vi "ParseSysexCapabilityQuery.vi"(8 "error in":errorcluster, 11 "Sysex Message":u8[](array[numeric]) format="%x") -> (0 "error out":errorcluster, 1 "IsValidSysex":bool, 3 "Board Pins":T1[](array[typedef]) {"Index"."DigitalIndex" step=1 format="D%d"; "Index"."AnalogIndex" min=0.0 step=1.0 format="A%#.0g"})   [LabVIEW 2020, in "FirmataClient.lvlib"]
doc: "Parse a message according to the Firmata Protocol Requirements. \n- https://github.com/firmata/protocol\n- https://github.com/firmata/protocol/blob/master/protocol.md"
uses:
  FirmataClient.lvlib
  controls/PinModesListData.ctl
  controls/PinModeData.ctl
  controls/FirmataPinModes.ctl
  controls/FGV-Mode.ctl
  controls/FirmataProtocolConstants.ctl
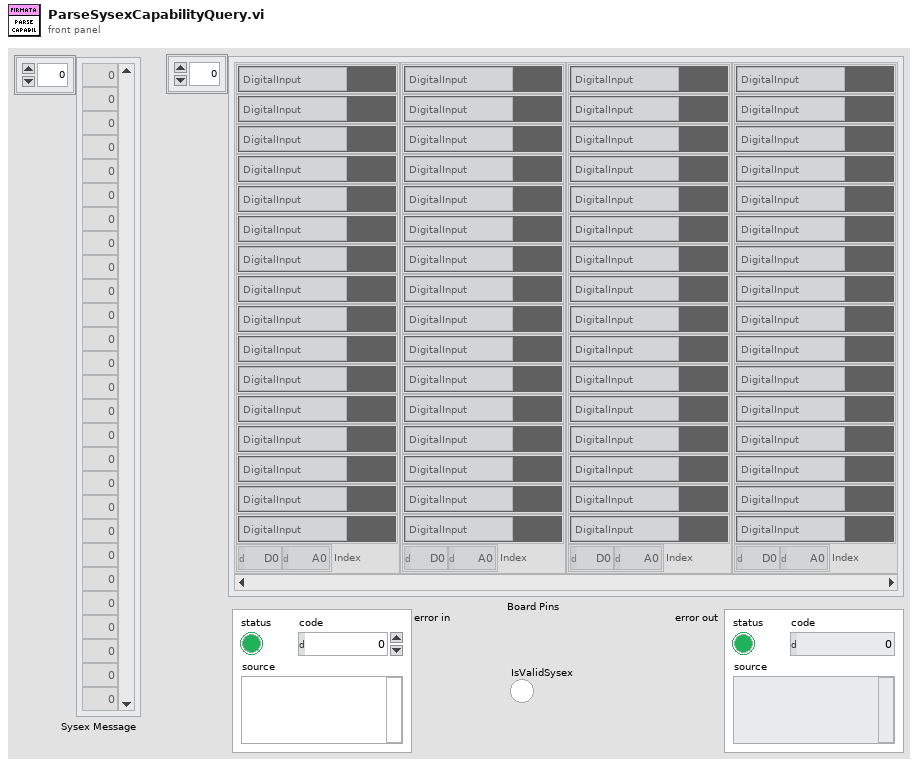
[diagram p1: front panel]
types:
  T1 = typedef "FirmataClient.lvlib/PinModesListData.ctl" = cluster{"DigitalInputMode":T2, "DigitalOutputMode":T2, "AnalogInputMode":T2, "PWMMode":T2, "ServoMode":T2, "ShiftMode":T2, "I2CMode":T2, "OneWireMode":T2, "StepperMode":T2, "EncoderMode":T2, "SerialMode":T2, "InputPullupMode":T2, "Ext.SPIMode":T2, "Ext.SonarMode":T2, "Ext.ToneMode":T2, "Ext.DHTMode":T2, "Index":cluster{"DigitalIndex":u16, "AnalogIndex":dbl}}
  T2 = typedef "FirmataClient.lvlib/PinModeData.ctl" = cluster{"Resolution":u8, "btn":bool, "PinMode":T3}
  T3 = typedef "FirmataClient.lvlib/FirmataPinModes.ctl" = enum16{"DigitalInput", "DigitalOutput", "AnalogInput", "PWM", "Servo", "Shift", "I2C", "OneWire", "Stepper", "Encoder", "Serial", "InputPullup", "Extended.SPI", "Extended.Sonar", "Extended.Tone", "Extended.DHT"}
  T4 = typedef "FirmataClient.lvlib/FirmataProtocolConstants.ctl" = u16
  T5 = typedef "FirmataClient.lvlib/FGV-Mode.ctl" = enum16{"Load Comport", "Load Board Capabilities", "Read"}
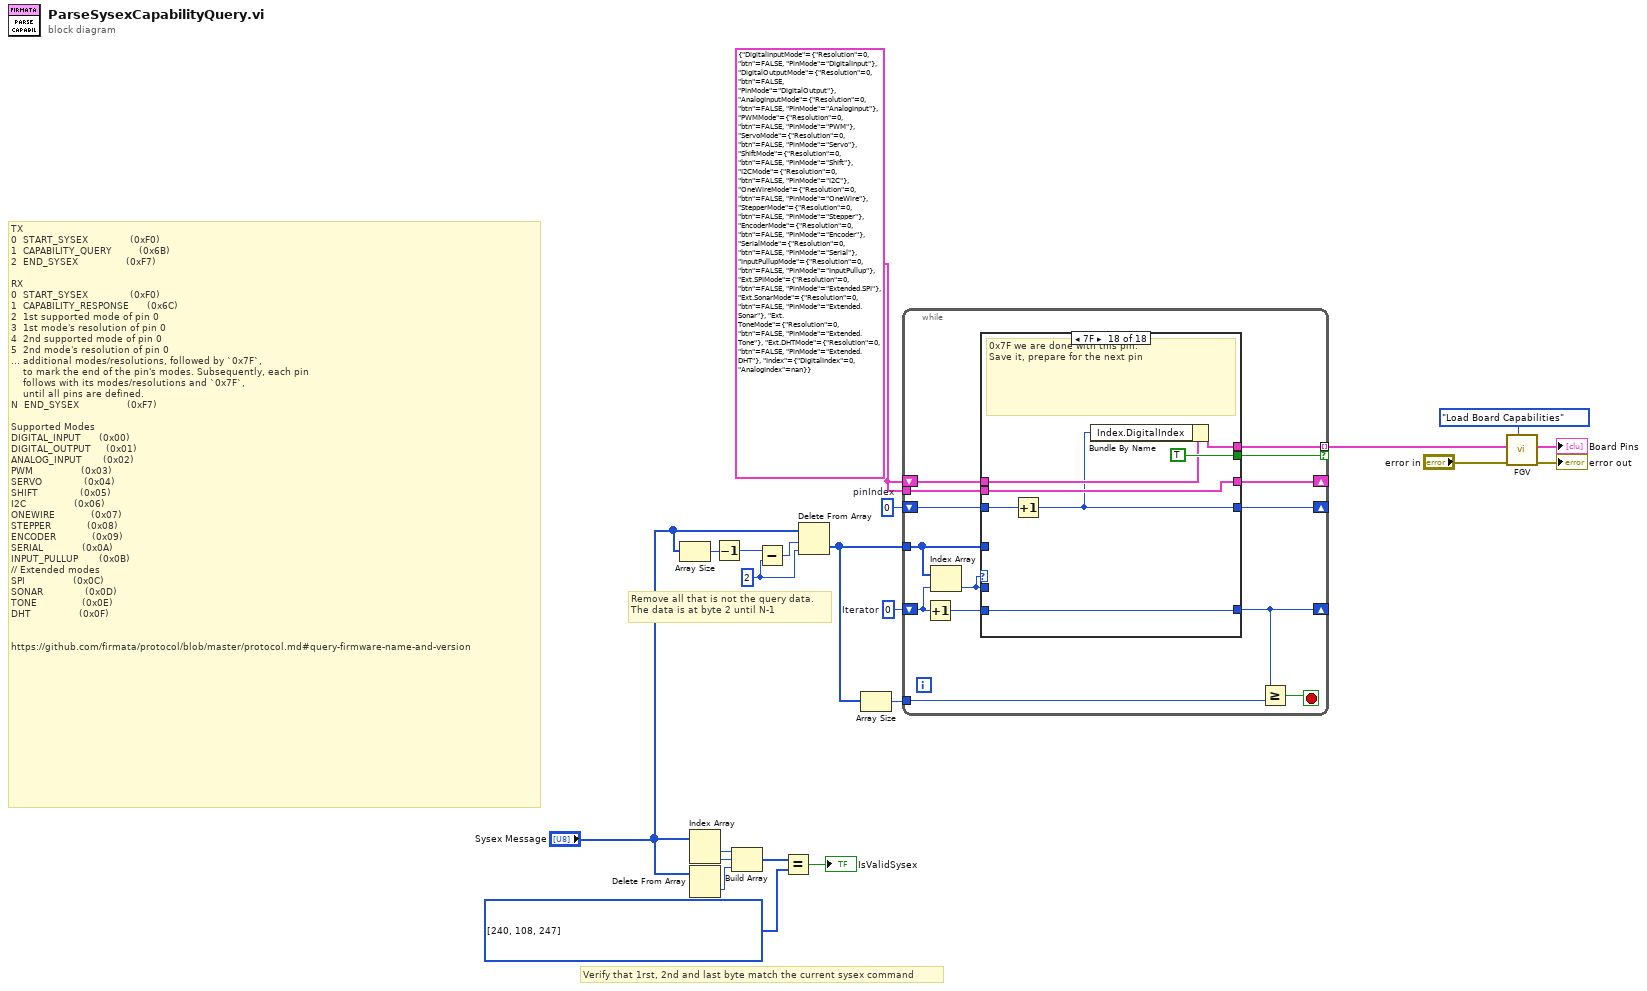
[diagram p0: block diagram]
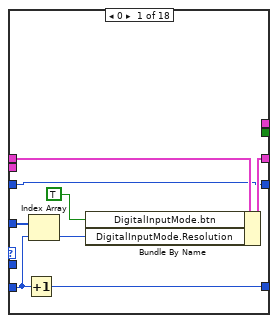
[diagram p2: hidden frame]
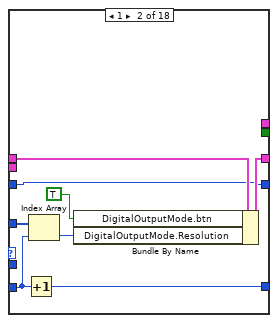
[diagram p3: hidden frame]
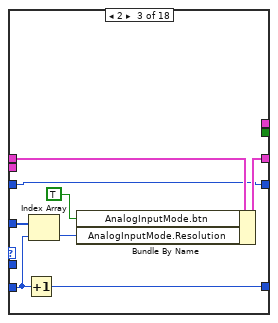
[diagram p4: hidden frame]
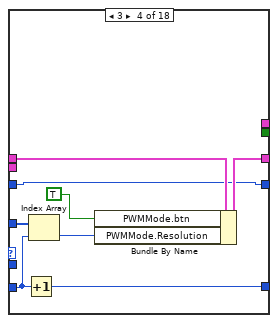
[diagram p5: hidden frame]
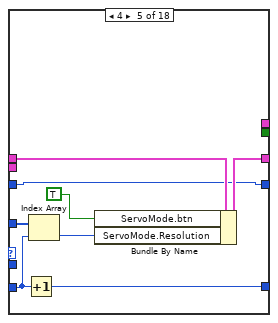
[diagram p6: hidden frame]
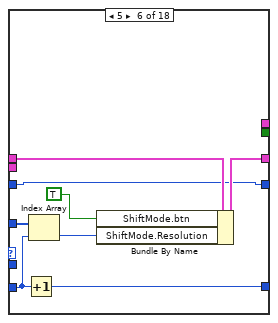
[diagram p7: hidden frame]
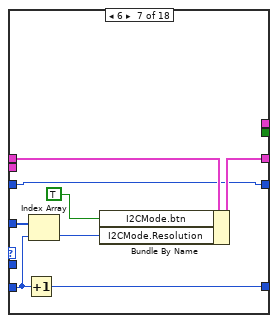
[diagram p8: hidden frame]
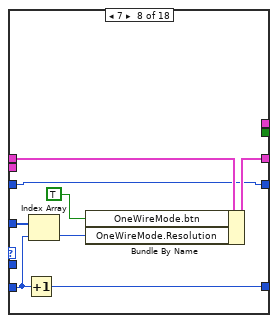
[diagram p9: hidden frame]
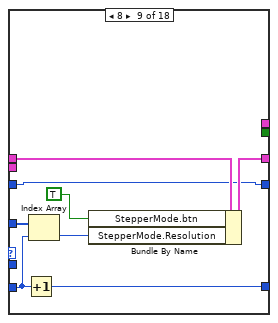
[diagram p10: hidden frame]
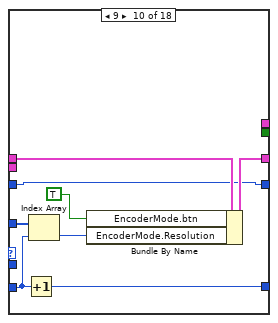
[diagram p11: hidden frame]
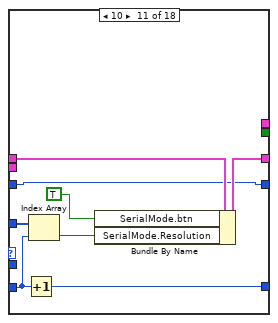
[diagram p12: hidden frame]
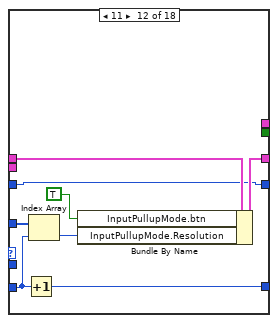
[diagram p13: hidden frame]
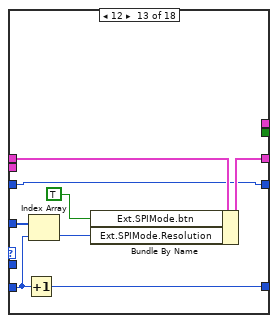
[diagram p14: hidden frame]
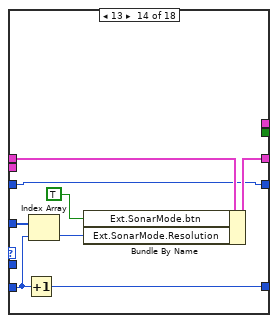
[diagram p15: hidden frame]
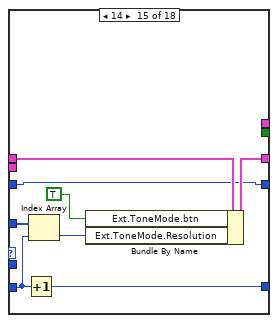
[diagram p16: hidden frame]
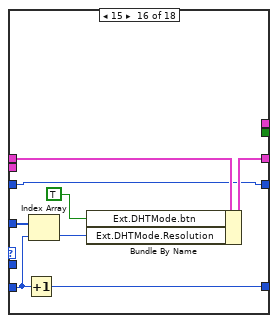
[diagram p17: hidden frame]
diagram:
  w3 = 0  # pinIndex
  w4 = T4[] [240, 108, 247] items=["ANALOG_IO_MESSAGE"=224, "DIGITAL_IO_MESSAGE"=144, "REPORT_ANALOG_PIN"=192, "REPORT_DIGITAL_PORT"=208, "START_SYSEX"=240, "END_SYSEX"=247, "SET_PIN_MODE"=244, "SET_DIGITAL_PIN_VALUE"=245, "PROTOCOL_VERSION"=249, "SYSTEM_RESET"=255, "SYSEX.EXTENDED_ID"=0, "SYSEX.RESERVED_USER_COMMANDs"=1, "SYSEX.ANALOG_MAPPING_QUERY"=105, "SYSEX.ANALOG_MAPPING_RESPONSE"=106, "SYSEX.CAPABILITY_QUERY"=107, "SYSEX.CAPABILITY_RESPONSE"=108, "SYSEX.PIN_STATE_QUERY"=109, "SYSEX.PIN_STATE_RESPONSE"=110, "SYSEX.REPORT_FIRMWARE"=121, "SYSEX.EXTENDED_ANALOG"=111, "SYSEX.STRING_DATA"=113, "SYSEX.REALTIME"=127, "SYSEX.NON_REALTIME"=126, "SYSEX.SAMPLING_INTERVAL"=122]
  w10 = 0  # Iterator
  w11 = T1 {"DigitalInputMode"={"Resolution"=0, "btn"=FALSE, "PinMode"=enum."DigitalInput"}, "DigitalOutputMode"={"Resolution"=0, "btn"=FALSE, "PinMode"=enum."DigitalOutput"}, "AnalogInputMode"={"Resolution"=0, "btn"=FALSE, "PinMode"=enum."AnalogInput"}, "PWMMode"={"Resolution"=0, "btn"=FALSE, "PinMode"=enum."PWM"}, "ServoMode"={"Resolution"=0, "btn"=FALSE, "PinMode"=enum."Servo"}, "ShiftMode"={"Resolution"=0, "btn"=FALSE, "PinMode"=enum."Shift"}, "I2CMode"={"Resolution"=0, "btn"=FALSE, "PinMode"=enum."I2C"}, "OneWireMode"={"Resolution"=0, "btn"=FALSE, "PinMode"=enum."OneWire"}, "StepperMode"={"Resolution"=0, "btn"=FALSE, "PinMode"=enum."Stepper"}, "EncoderMode"={"Resolution"=0, "btn"=FALSE, "PinMode"=enum."Encoder"}, "SerialMode"={"Resolution"=0, "btn"=FALSE, "PinMode"=enum."Serial"}, "InputPullupMode"={"Resolution"=0, "btn"=FALSE, "PinMode"=enum."InputPullup"}, "Ext.SPIMode"={"Resolution"=0, "btn"=FALSE, "PinMode"=enum."Extended.SPI"}, "Ext.SonarMode"={"Resolution"=0, "btn"=FALSE, "PinMode"=enum."Extended.Sonar"}, "Ext.ToneMode"={"Resolution"=0, "btn"=FALSE, "PinMode"=enum."Extended.Tone"}, "Ext.DHTMode"={"Resolution"=0, "btn"=FALSE, "PinMode"=enum."Extended.DHT"}, "Index"={"DigitalIndex"=0, "AnalogIndex"=nan}}
  w14 = 2 ("index")
  # "Remove all that is not the query data. \nThe data is at byte 2 until N-1"
  # "Verify that 1rst, 2nd and last byte match the current sysex command"
  # "TX\n0  START_SYSEX              (0xF0)\n1  CAPABILITY_QUERY         (0x6B)\n2  END_SYSEX                (0xF7)\n\nRX\n0  START_SYSEX              (0xF0)\n1  CAPABILITY_RESPONSE      (0x6C)\n2  1st supported mode of pin 0\n3  1st mode's resolution of pin 0\n4  2nd supported mode of pin 0\n5  2nd mode's resolution of pin 0\n... additional modes/resolutions, followed by `0x7F`,\n    to mark the end of the pin's modes. Subsequently, each pin\n    follows with its modes/resolutions and `0x7F`,\n    until all pins are defined.\nN  END_SYSEX                (0xF7)\n\nSupported Modes\nDIGITAL_INPUT      (0x00)\nDIGITAL_OUTPUT     (0x01)\nANALOG_INPUT       (0x02)\nPWM                (0x03)\nSERVO              (0x04)\nSHIFT              (0x05)\nI2C                (0x06)\nONEWIRE            (0x07)\nSTEPPER            (0x08)\nENCODER            (0x09)\nSERIAL             (0x0A)\nINPUT_PULLUP       (0x0B)\n// Extended modes \nSPI                (0x0C)\nSONAR              (0x0D)\nTONE               (0x0E)\nDHT                (0x0F)\n\n\nhttps://github.com/firmata/protocol/blob/master/protocol.md#query-firmware-name-and-version"
  n1 = Array Size(array="Sysex Message") -> (size(s)=w16:i32)
  n2 = Index Array(array="Sysex Message") -> (element #1=w21:u8, element #2=w19:u8)  [unwired: 2 in]
  n3 = Delete From Array(array="Sysex Message") -> (deleted portion=w20:u8)  [unwired: 2 in, 1 out]
  n4 = Decrement(x=w16) -> (x-1=w15:i32)
  n5 = Build Array(w21, w19, w20) -> (w18:u8[])
  n6 = Subtract(x=w15, y=w14) -> (x-y=w13:i32)
  n7 = Equal?(x=w18, y=w4) -> (x = y?=→"IsValidSysex":bool)
  n8 = Delete From Array(array="Sysex Message", length=w13, index=w14) -> (deleted portion=w9:u8[])  [unwired: 1 out]
  n9 = Array Size(array=w9) -> (size(s)=w8:i32)
  n10 = while {
    tunnel: w11 -> [w30]
    shift-right: [w31] -> _
    shift-left: w11 -> [w29]
    tunnel: w9 -> [w33]
    shift-right: [w26] -> _
    shift-left: w10 -> [w35]
    tunnel: [w28] -> w6 mode=indexing if=w27
    tunnel: w8 -> [w24]
    shift-right: [w22] -> _
    shift-left: w3 -> [w23]
    stop <- w25 stop-if-true
    n11 = Increment(x=w35) -> (x+1=w34:i32)
    n12 = Index Array(array=w33, index=w35) -> (element=w32:u8)
    n13 = case shown="7F" w32 {
      tunnel: w34 -> [w40 w48 w56 w64 w72 w80 w88 w96 w104 w112 w120 w128 w136 w144 w152 w160 w165 w169]
      tunnel: w33 -> [w43 w51 w59 w67 w75 w83 w91 w99 w107 w115 w123 w131 w139 w147 w155 w163 _ _]
      tunnel: w32 -> [_ _ _ _ _ _ _ _ _ _ _ _ _ _ _ _ _ _]
      tunnel: [w41 w49 w57 w65 w73 w81 w89 w97 w105 w113 w121 w129 w137 w145 w153 w161 w166 w173] -> w31
      tunnel: w30 -> [_ _ _ _ _ _ _ _ _ _ _ _ _ _ _ _ _ w173]
      tunnel: w29 -> [w42 w50 w58 w66 w74 w82 w90 w98 w106 w114 w122 w130 w138 w146 w154 w162 w166 w171]
      tunnel: [_ _ _ _ _ _ _ _ _ _ _ _ _ _ _ _ _ w170] -> w28
      tunnel: [_ _ _ _ _ _ _ _ _ _ _ _ _ _ _ _ _ TRUE] -> w27
      tunnel: [w39 w47 w55 w63 w71 w79 w87 w95 w103 w111 w119 w127 w135 w143 w151 w159 w165 w169] -> w26
      tunnel: w23 -> [w36 w44 w52 w60 w68 w76 w84 w92 w100 w108 w116 w124 w132 w140 w148 w156 w164 w168]
      tunnel: [w36 w44 w52 w60 w68 w76 w84 w92 w100 w108 w116 w124 w132 w140 w148 w156 w164 w167] -> w22
      frame 0 {
        n14 = Increment(x=w40) -> (x+1=w39:i32)
        n15 = Index Array(array=w43, index=w40) -> (element=w38:u8)
        n16 = Bundle By Name(cluster=w42, "DigitalInputMode.btn"=TRUE ("btn"), "DigitalInputMode.Resolution"=w38) -> (w41:T1)
      }
      frame 1 {
        n17 = Increment(x=w48) -> (x+1=w47:i32)
        n18 = Index Array(array=w51, index=w48) -> (element=w46:u8)
        n19 = Bundle By Name(cluster=w50, "DigitalOutputMode.btn"=TRUE ("btn"), "DigitalOutputMode.Resolution"=w46) -> (w49:T1)
      }
      frame 2 {
        n20 = Increment(x=w56) -> (x+1=w55:i32)
        n21 = Index Array(array=w59, index=w56) -> (element=w54:u8)
        n22 = Bundle By Name(cluster=w58, "AnalogInputMode.btn"=TRUE ("btn"), "AnalogInputMode.Resolution"=w54) -> (w57:T1)
      }
      frame 3 {
        n23 = Increment(x=w64) -> (x+1=w63:i32)
        n24 = Index Array(array=w67, index=w64) -> (element=w62:u8)
        n25 = Bundle By Name(cluster=w66, "PWMMode.btn"=TRUE ("btn"), "PWMMode.Resolution"=w62) -> (w65:T1)
      }
      frame 4 {
        n26 = Increment(x=w72) -> (x+1=w71:i32)
        n27 = Index Array(array=w75, index=w72) -> (element=w70:u8)
        n28 = Bundle By Name(cluster=w74, "ServoMode.btn"=TRUE ("btn"), "ServoMode.Resolution"=w70) -> (w73:T1)
      }
      frame 5 {
        n29 = Increment(x=w80) -> (x+1=w79:i32)
        n30 = Index Array(array=w83, index=w80) -> (element=w78:u8)
        n31 = Bundle By Name(cluster=w82, "ShiftMode.btn"=TRUE ("btn"), "ShiftMode.Resolution"=w78) -> (w81:T1)
      }
      frame 6 {
        n32 = Increment(x=w88) -> (x+1=w87:i32)
        n33 = Index Array(array=w91, index=w88) -> (element=w86:u8)
        n34 = Bundle By Name(cluster=w90, "I2CMode.btn"=TRUE ("btn"), "I2CMode.Resolution"=w86) -> (w89:T1)
      }
      frame 7 {
        n35 = Increment(x=w96) -> (x+1=w95:i32)
        n36 = Index Array(array=w99, index=w96) -> (element=w94:u8)
        n37 = Bundle By Name(cluster=w98, "OneWireMode.btn"=TRUE ("btn"), "OneWireMode.Resolution"=w94) -> (w97:T1)
      }
      frame 8 {
        n38 = Increment(x=w104) -> (x+1=w103:i32)
        n39 = Index Array(array=w107, index=w104) -> (element=w102:u8)
        n40 = Bundle By Name(cluster=w106, "StepperMode.btn"=TRUE ("btn"), "StepperMode.Resolution"=w102) -> (w105:T1)
      }
      frame 9 {
        n41 = Increment(x=w112) -> (x+1=w111:i32)
        n42 = Index Array(array=w115, index=w112) -> (element=w110:u8)
        n43 = Bundle By Name(cluster=w114, "EncoderMode.btn"=TRUE ("btn"), "EncoderMode.Resolution"=w110) -> (w113:T1)
      }
      frame 10 {
        n44 = Increment(x=w120) -> (x+1=w119:i32)
        n45 = Index Array(array=w123, index=w120) -> (element=w118:u8)
        n46 = Bundle By Name(cluster=w122, "SerialMode.btn"=TRUE ("btn"), "SerialMode.Resolution"=w118) -> (w121:T1)
      }
      frame 11 {
        n47 = Increment(x=w128) -> (x+1=w127:i32)
        n48 = Index Array(array=w131, index=w128) -> (element=w126:u8)
        n49 = Bundle By Name(cluster=w130, "InputPullupMode.btn"=TRUE ("btn"), "InputPullupMode.Resolution"=w126) -> (w129:T1)
      }
      frame 12 {
        n50 = Increment(x=w136) -> (x+1=w135:i32)
        n51 = Index Array(array=w139, index=w136) -> (element=w134:u8)
        n52 = Bundle By Name(cluster=w138, "Ext.SPIMode.btn"=TRUE ("btn"), "Ext.SPIMode.Resolution"=w134) -> (w137:T1)
      }
      frame 13 {
        n53 = Increment(x=w144) -> (x+1=w143:i32)
        n54 = Index Array(array=w147, index=w144) -> (element=w142:u8)
        n55 = Bundle By Name(cluster=w146, "Ext.SonarMode.btn"=TRUE ("btn"), "Ext.SonarMode.Resolution"=w142) -> (w145:T1)
      }
      frame 14 {
        n56 = Increment(x=w152) -> (x+1=w151:i32)
        n57 = Index Array(array=w155, index=w152) -> (element=w150:u8)
        n58 = Bundle By Name(cluster=w154, "Ext.ToneMode.btn"=TRUE ("btn"), "Ext.ToneMode.Resolution"=w150) -> (w153:T1)
      }
      frame 15 {
        n59 = Increment(x=w160) -> (x+1=w159:i32)
        n60 = Index Array(array=w163, index=w160) -> (element=w158:u8)
        n61 = Bundle By Name(cluster=w162, "Ext.DHTMode.btn"=TRUE ("btn"), "Ext.DHTMode.Resolution"=w158) -> (w161:T1)
      }
      frame Default {
      }
      frame 127 {
        # "0x7F we are done with this pin.\nSave it, prepare for the next pin"
        n62 = Increment(x=w168) -> (x+1=w167:i32)
        n63 = Bundle By Name(cluster=w171, "Index.DigitalIndex"=w167) -> (w170:T1)
      }
    }
    n64 = Greater Or Equal?(x=w26, y=w24) -> (x >= y?=w25:bool)
  }
  n65 = call "FGV.vi"("Mode"=FGV-Mode."Load Board Capabilities", "error in"="error in", "Board Pins In"=w6) -> ("error out"=→"error out":errorcluster, "Board Pins Out"=→"Board Pins":T1[])  [unwired: 6 in, 1 out]
